vi "create.vi"(6 "Type":enum16{"INFO", "FLAG", "ERROR", "SUCCESS"}(ring), 7 "Time Stamp (now)":timestamp format="%<%x %.3X>T", 8 "error in":errorcluster, 9 "Name":string, 10 "assets":refnum<class "asset.lvclass">[](array[class]), 11 "Nominal Client in":refnum<class "Nominal Client.lvclass">) -> (0 "error out":errorcluster, 3 "event":refnum<class "event.lvclass">)   [LabVIEW 2020, in "event.lvclass"]
uses:
  event.lvclass
  Nominal Client/Nominal Client.lvclass
  asset/asset.lvclass
  event.lvclass/event.ctl
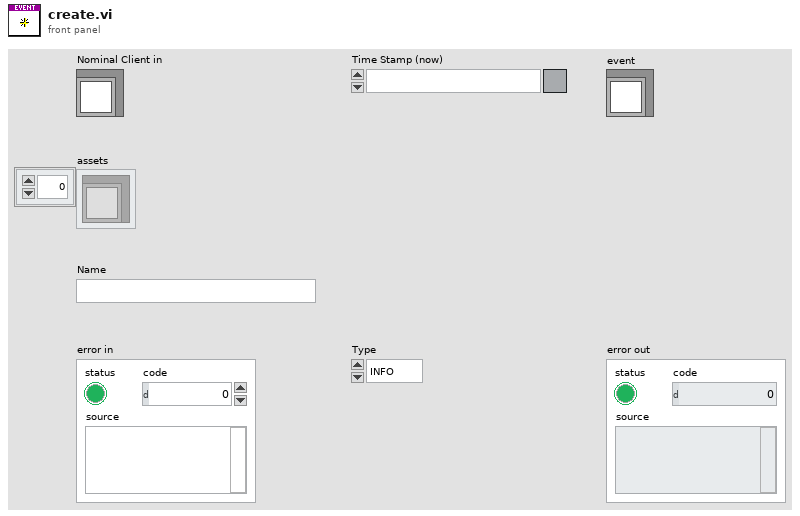
[diagram p1: front panel]
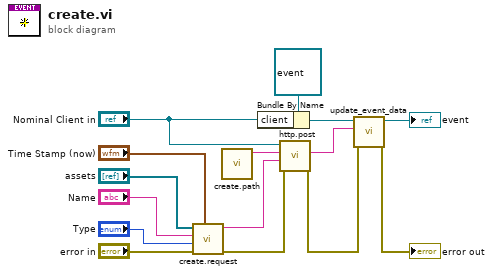
[diagram p0: block diagram]
diagram:
  n1 = call "create.request.vi"("Time Stamp (now: system time)"="Time Stamp (now)", "error in"="error in", "Type"="Type", "Name"="Name", "assets"="assets") -> ("error out"=w12:errorcluster, "request"=w13:string)  [unwired: 5 in]
  n2 = call "create.path.vi"() -> ("path"=w15:string)  [unwired: 11 in]
  n3 = Bundle By Name(cluster=refnum<class "event.lvclass"> refnum ("event in"), "client"="Nominal Client in") -> (w6:refnum<class "event.lvclass">)
  n4 = call "http.post.vi"("error in"=w12, "Request body"=w13, "Path"=w15, "Nominal Client in"="Nominal Client in") -> ("error out"=w2:errorcluster, "Response"=w5:string)  [unwired: 4 in, 2 out]
  n5 = call "update_event_data.vi"("error in"=w2, "JSON"=w5, "event in"=w6) -> ("error out"=→"error out":errorcluster, "event out"=→"event":refnum<class "event.lvclass">)  [unwired: 7 in]
